vi "GetDioIn.vi"(11 "error in":errorcluster caption="错误输入") -> (0 "DIO":bool[](array[boolean]), 1 "DIO":u8, 3 "error out":errorcluster caption="错误输出")   [LabVIEW 2016]
uses:
  PLC-Lab/lib/gusb.dll
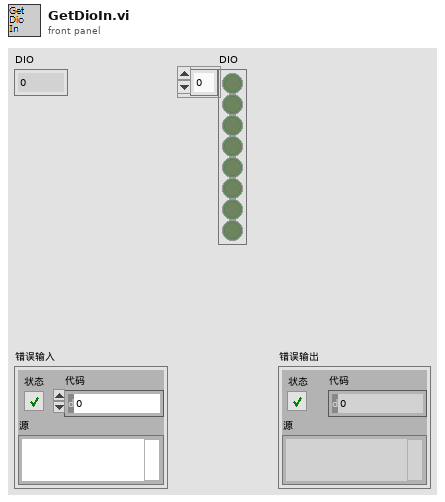
[diagram p1: front panel]
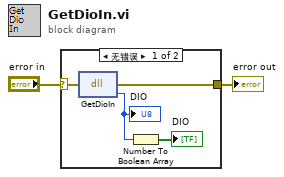
[diagram p0: block diagram]
diagram:
  n1 = case shown="无错误" "error in" {
    selector: "error in" -> [w6 w7]
    tunnel: [w5 w7] -> w1
    frame No Error {
      n2 = dll-call lib="E:/Camproject/2018/2018.1Labview/PLC-Lab/lib/gusb.dll" fn="GetDioIn"(error in=w6) -> (error out=w5:errorcluster, "DIO"=w4:u8)  [unwired: 2 in, 1 out]
      "DIO" <- w4
      n3 = Number To Boolean Array(number=w4) -> (Boolean array=→"DIO":bool[])
    }
    frame Error {
    }
  }
  "error out" <- w1
